vi "GetNewKeyPress.vi"(0 "n Array":dbl[](array[numeric]), 1 "n+1 Array":dbl[](array[numeric])) -> (2 "Extracted Different":dbl=-1.0, 3 "Extracted Index":i32, 4 "Changes?":bool)   [LabVIEW 2015]
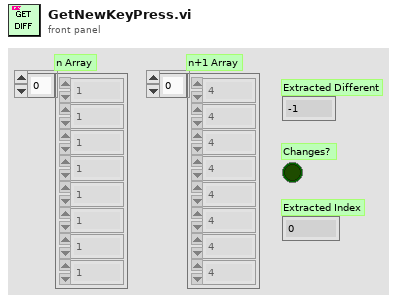
[diagram p1: front panel]
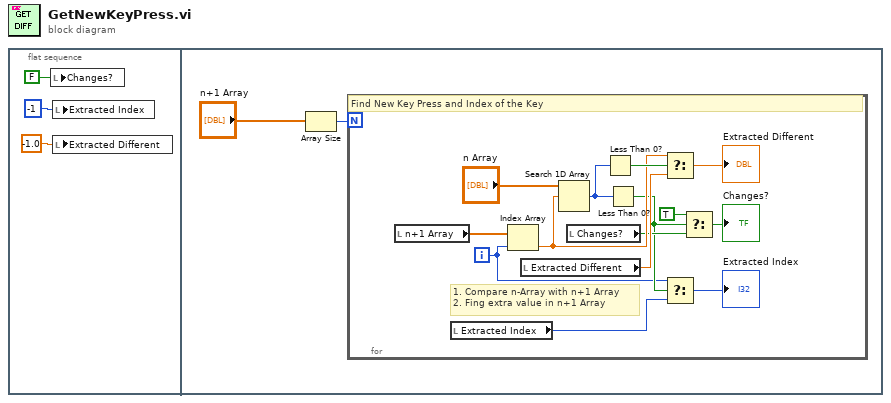
[diagram p0: block diagram]
diagram:
  n1 = flat-sequence {
    frame #0 {
      n2 = local write "Changes?"(FALSE ("Changes?")) -> ()
      n3 = local write "Extracted Index"(-1 ("Extracted Index")) -> ()
      n4 = local write "Extracted Different"(-1.0 ("Extracted Different")) -> ()
    }
    frame #1 {
      n5 = Array Size(array="n+1 Array") -> (size(s)=w4:i32)
      n6 = for {
        N: w4 -> [_]
        i -> [w8]
        # "1. Compare n-Array with n+1 Array\n2. Fing extra value in n+1 Array"
        # "Find New Key Press and Index of the Key"
        n7 = local read "n+1 Array"() -> (w18:dbl[])
        n8 = local read "Extracted Index"() -> (w6:i32)
        n9 = Index Array(array=w18, index=w8) -> (element=w16:dbl)
        n10 = local read "Extracted Different"() -> (w14:dbl)
        n11 = Search 1D Array(1D array="n Array", element=w16) -> (index of element=w13:i32)  [unwired: 1 in]
        n12 = local read "Changes?"() -> (w10:bool)
        n13 = Less Than 0?(x=w13) -> (x < 0?=w17:bool)
        n14 = Less Than 0?(x=w13) -> (x < 0?=w9:bool)
        n15 = Select(t=w16, s=w17, f=w14) -> (s? t:f=→"Extracted Different":dbl)
        n16 = Select(t=w8, s=w9, f=w6) -> (s? t:f=→"Extracted Index":i32)
        n17 = Select(t=TRUE, s=w9, f=w10) -> (s? t:f=→"Changes?":bool)
      }
    }
  }
